vi "Exemple structure condition.vi"() -> ()   [LabVIEW 2014]
panel:
  in  "stop":bool
  out "String":string
  in  "number 2":dbl
  in  "number 1":dbl
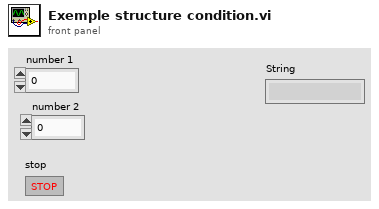
[diagram p1: front panel]
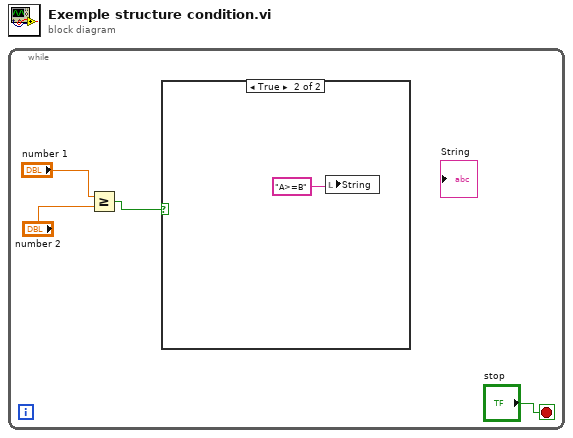
[diagram p0: block diagram]
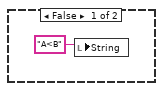
[diagram p2: hidden frame]
diagram:
  n1 = while {
    stop <- "stop" stop-if-true
    n2 = Greater Or Equal?(x="number 1", y="number 2") -> (x >= y?=w2:bool)
    n3 = case shown="True" w2 {
      frame False {
        n4 = local write "String"("A<B") -> ()
      }
      frame True {
        n5 = local write "String"("A>=B") -> ()
      }
    }
  }
